vi "readTemperature.vi"(8 "error in (no error)":errorcluster, 9 "TemperatureType":T1, 10 "id":T2=1, 11 "CoolerControler in":refnum<class "CoolerControler.lvclass">) -> (0 "error out":errorcluster, 2 "temperature":sgl, 3 "CoolerControler out":refnum<class "CoolerControler.lvclass">)   [LabVIEW 2016, in "CoolerControler.lvclass"]
uses:
  CoolerControler.lvclass
  typedefs/CoolerId.ctl
  typedefs/readTempreature.ctl
  SerialCommand/CoolerSerialCommand.lvclass
  typedefs/dataUnit.ctl
  typedefs/CoolerQuery.ctl
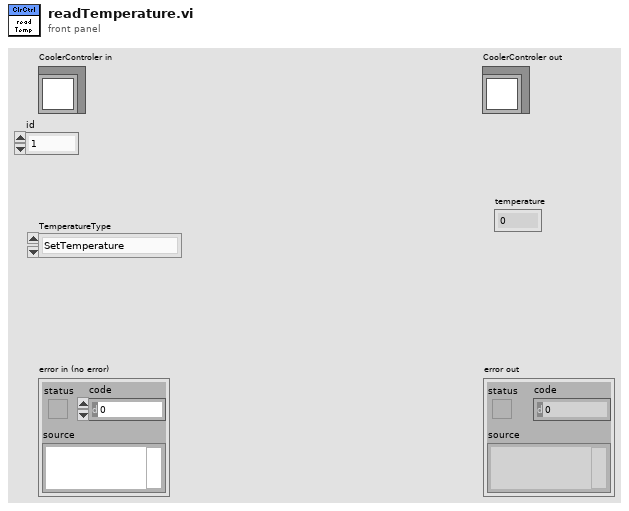
[diagram p1: front panel]
types:
  T1 = typedef "readTempreature.ctl" = enum16{"SetTemperature", "AmbientTemperature", "SupplyTemperature", "ExternalRTDTemperature", "ReturnTemperature", "ExternalThermistor"}
  T2 = typedef "CoolerId.ctl" = u16
  T3 = typedef "dataUnit.ctl" = enum16{"temperature", "flow", "current", "PID", "fanSpeed", "time", "PWM", "TEDriveLevel", "Number"}
  T4 = typedef "CoolerQuery.ctl" = enum16{"ReadSerialWatchdog", "ReadControlSensor", "ReadSetTemperature", "ReadSupplyTemperature", "ReadExternalRTD", "ReadExternalThermistor", "ReadReturnTemperature", "ReadAmbientTemperature", "ReadProcessFlow", "ReadTECBank1Current", "ReadTECBank2Current", "ReadTEDriveLevel", "ReadAlarmStateLevel1", "ReadAlarmStateLevel21", "ReadAlarmStateLevel22", "ReadWarningStateLevel1", "ReadHighSupplyTempWarning", "ReadLowSupplyTempWarning", "ReadHighAmbientTempWarning", "ReadLowAmbientTempWarning", "ReadLowProcessFlowWarning", "ReadHighSupplyTempAlarm", "ReadLowSupplyTempAlarm", "ReadHighAmbientTempAlarm", "ReadLowAmbientTempAlarm", "ReadLowProcessFlowAlarm", "ReadPWMandRelayStatus", "ReadPIDStatus", "ReadUnitUpTime", "ReadFan1Speed", "ReadFan2Speed", "ReadFan3Speed", "ReadFan4Speed"}
  T5 = typedef "response.ctl" = cluster{"deviceId":string, "commandNumber":string, "errorActive":bool, "commandName":string, "responseData":string, "checkSum":string}
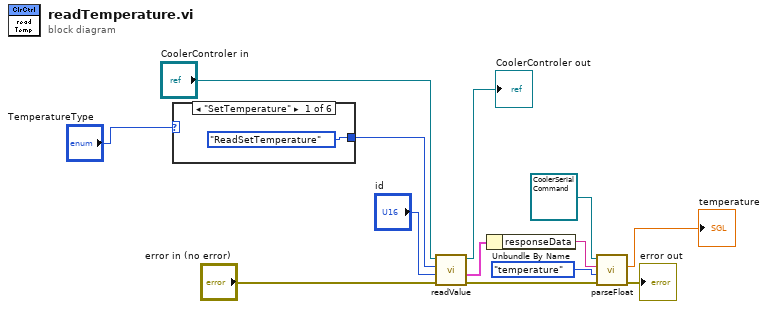
[diagram p0: block diagram]
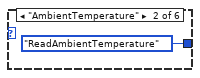
[diagram p2: hidden frame]
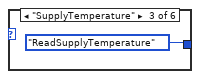
[diagram p3: hidden frame]
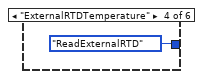
[diagram p4: hidden frame]
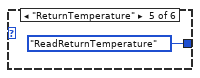
[diagram p5: hidden frame]
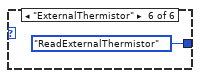
[diagram p6: hidden frame]
diagram:
  n1 = case shown="\"SetTemperature\"" "TemperatureType" {
    tunnel: [CoolerQuery."ReadSetTemperature" ("CoolerQuery") CoolerQuery."ReadAmbientTemperature" ("CoolerQuery") CoolerQuery."ReadSupplyTemperature" ("CoolerQuery") CoolerQuery."ReadExternalRTD" ("CoolerQuery") CoolerQuery."ReadReturnTemperature" ("CoolerQuery") CoolerQuery."ReadExternalThermistor" ("CoolerQuery")] -> w10
    frame "SetTemperature" {
    }
    frame "AmbientTemperature" {
    }
    frame "SupplyTemperature" {
    }
    frame "ExternalRTDTemperature" {
    }
    frame "ReturnTemperature" {
    }
    frame "ExternalThermistor" {
    }
  }
  n2 = call "readValue.vi"("error in (no error)"="error in (no error)", "id"="id", "CoolerQuery"=w10, "CoolerControler in"="CoolerControler in") -> ("error out"=w6:errorcluster, "response out"=w8:T5, "CoolerControler out"=→"CoolerControler out":refnum<class "CoolerControler.lvclass">)  [unwired: 4 in, 1 out]
  n3 = Unbundle By Name(w8) -> ("responseData"=w7:string)
  n4 = call "parseFloat.vi"("error in (no error)"=w6, "unit"=dataUnit."temperature", "commandData"=w7, "CoolerSerialCommand in"=refnum<class "CoolerSerialCommand.lvclass"> refnum) -> ("error out"=→"error out":errorcluster, "value"=→"temperature":sgl)  [unwired: 4 in, 2 out]
